vi "GetOutputWireBranches.vi"(6 "error in":errorcluster, 9 "FlatSequenceFrame in":refnum<class "FlatSequenceFrame.lvclass">) -> (0 "error out":errorcluster, 3 "FlatSequenceFrame out":refnum<class "FlatSequenceFrame.lvclass">, 4 "branches":string[](array[string]))   [LabVIEW 2014, in "Raspberry Pi Compatible Compiler for LabVIEW.lvlib" / "FlatSequenceFrame.lvclass"]
uses:
  FlatSequenceFrame.lvclass
  FlatSequenceFrame.lvclass/FlatSequenceFrame.ctl
  FlatSequenceOuterTunnel/FlatSequenceOuterTunnel.lvclass
  FlatSequenceInnerTunnel/FlatSequenceInnerTunnel.lvclass
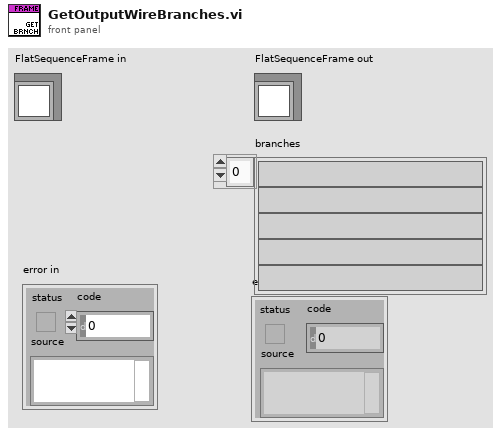
[diagram p1: front panel]
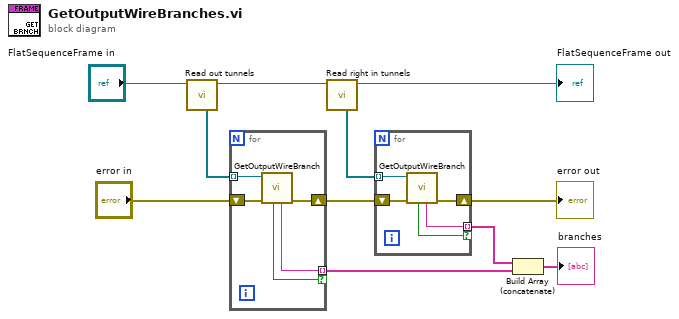
[diagram p0: block diagram]
diagram:
  n1 = call "Read out tunnels.vi"("FlatSequenceFrame in"="FlatSequenceFrame in") -> ("FlatSequenceFrame out"=w10:refnum<class "FlatSequenceFrame.lvclass">, "out tunnels"=w8:refnum<class "FlatSequenceOuterTunnel.lvclass">[])  [unwired: 7 in]
  n2 = for {
    tunnel: w8 -> [w16] mode=indexing
    shift-right: [w14] -> w9
    shift-left: "error in" -> [w15]
    tunnel: [w13] -> w4 mode=indexing if=w12
    n3 = call-dynamic "GetOutputWireBranch.vi"("error in"=w15, "Tunnel in"=w16) -> ("error out"=w14:errorcluster, "branches"=w13:string, "branched"=w12:bool)  [unwired: 4 in, 1 out]
  }
  n4 = call "Read right in tunnels.vi"("FlatSequenceFrame in"=w10) -> ("FlatSequenceFrame out"=→"FlatSequenceFrame out":refnum<class "FlatSequenceFrame.lvclass">, "right in tunnels"=w11:refnum<class "FlatSequenceInnerTunnel.lvclass">[])  [unwired: 7 in]
  n5 = for {
    tunnel: w11 -> [w21] mode=indexing
    shift-right: [w19] -> w1
    shift-left: w9 -> [w20]
    tunnel: [w18] -> w5 mode=indexing if=w17
    n6 = call-dynamic "GetOutputWireBranch.vi"("error in"=w20, "Tunnel in"=w21) -> ("error out"=w19:errorcluster, "branches"=w18:string, "branched"=w17:bool)  [unwired: 4 in, 1 out]
  }
  "error out" <- w1
  n7 = Build Array (concatenate)(w5, w4) -> (→"branches":string[])
